vi "GetCameraData.vi"(8 "error in (no error)":errorcluster, 11 "3D Scene in":refnum<class "3D Scene.lvclass">) -> (0 "error out":errorcluster)   [LabVIEW 2009]
uses:
  3D Scene.lvclass
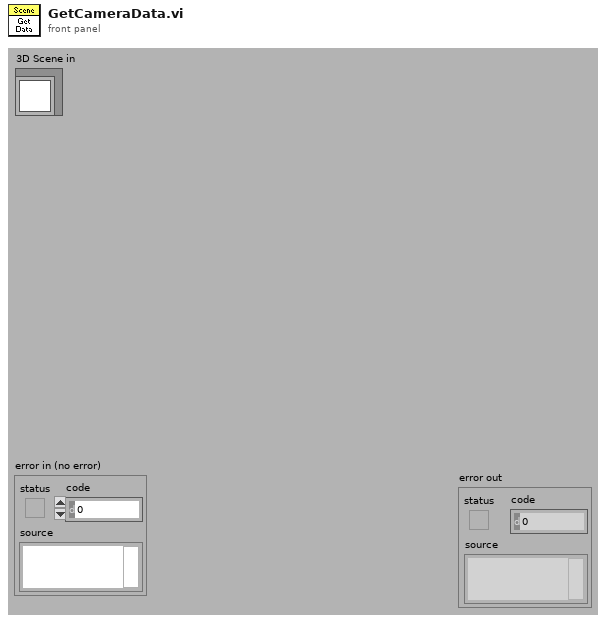
[diagram p1: front panel]
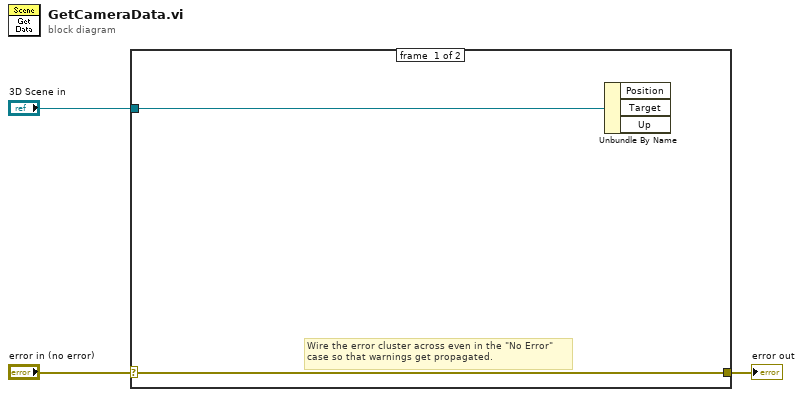
[diagram p0: block diagram]
diagram:
  n1 = case shown="No Error" "error in (no error)" {
    selector: "error in (no error)" -> [w5 w6]
    tunnel: [w5 w6] -> w2
    tunnel: "3D Scene in" -> [w4 _]
    frame #0 {
      # "Wire the error cluster across even in the \"No Error\"\ncase so that warnings get propagated."
      n2 = Unbundle By Name(w4) -> ()  [unwired: 3 out]
    }
    frame #1 {
    }
  }
  "error out" <- w2
